vi "GetMeasDataTag.vi"(10 "channel id":string, 11 "tags":T1[](array[typedef])) -> (3 "measurement data tag":T1)   [LabVIEW 2017, in "DeviceModelHelpers.lvlib"]
doc: "Returns the measurement data tag for the channel specified by the channel ID."
uses:
  <vilib>/addons/InsightCM/Utilities/DeviceModelHelpers/DeviceModelHelpers.lvlib
  <vilib>/addons/InsightCM/MessageBus/Base/controls/Tag.ctl
  <vilib>/addons/InsightCM/MessageBus/Base/controls/KeyValuePair.ctl
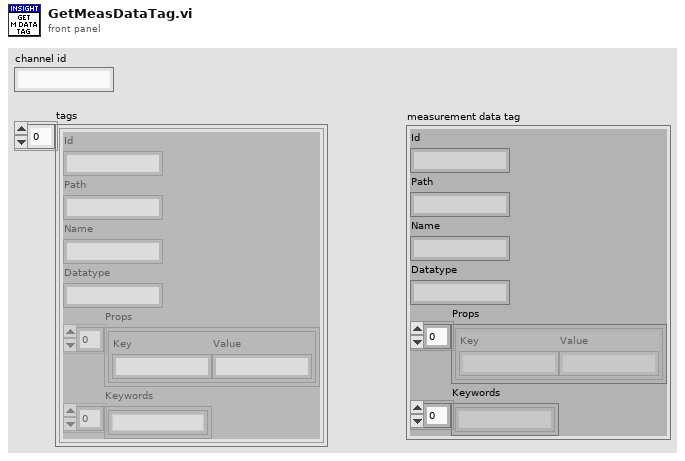
[diagram p1: front panel]
types:
  T1 = typedef "Tag.ctl" = cluster{"Id":string, "Path":string, "Name":string, "Datatype":string, "Props":T2[], "Keywords":string[]}
  T2 = typedef "KeyValuePair.ctl" = cluster{"Key":string, "Value":string}
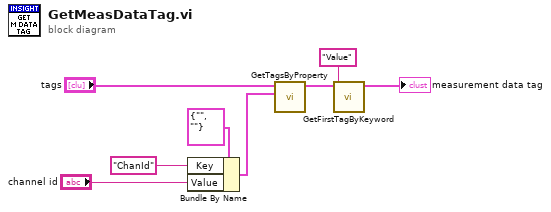
[diagram p0: block diagram]
diagram:
  n1 = Bundle By Name(cluster=T2 {"Key"="", "Value"=""} ("property"), "Key"="ChanId", "Value"="channel id") -> (w2:T2)
  n2 = call <vilib>:"GetTagsByProperty.vi"("property"=w2, "tags"="tags") -> ("matches"=w7:T1[])  [unwired: 9 in]
  n3 = call <vilib>:"GetFirstTagByKeyword.vi"("keyword"="Value", "tags"=w7) -> ("first tag"=→"measurement data tag":T1)  [unwired: 9 in]
